vi "PH_BackreflectionMeas.ProcCases.vi"(0 "i ref in":refnum<vi>, 1 "selector":string, 2 "Data":T1, 3 "call cluster":T2={"Object"="", "Selector"="", "CallType"=enum."synchronous", "Async Object"="", "Async Selector"="", "Data Descriptor"="", "Data"=[], "Error #"=0, "Expire"=0}, 5 "error in (no error)":errorcluster) -> (14 "i ref out":refnum<vi>, 17 "answer cluster":T2={"Object"="", "Selector"="", "CallType"=enum."synchronous", "Async Object"="", "Async Selector"="", "Data Descriptor"="", "Data"=[], "Error #"=0, "Expire"=0}, 19 "error out":errorcluster)   [LabVIEW 2014, in "PH_BackreflectionMeas.lvlib"]
doc: "This method is called by a process from within the default case in the event loop. The methods of a class that are linked to events will be called from THIS method. Add your code here."
uses:
  PH_BackreflectionMeas.lvlib
  CS_Core/CSSystem/CoreDefs/CoreDefs.call_type.ctl
  CS_Core/BaseProcess/BaseProcess.descriptor string definition.ctl
  CS_Core/CSSystem/CoreDefs/CoreDefs.rawDataType.ctl
  PH_Basics/PH_StatusHandler/PH_StatusHandler.Status.ctl
  CS_Core/CSSystem/CoreLib/CoreLib.string 2 byte array.vi
  CS_Core/BaseProcess/BaseProcess.lvlib
  CS_Core/CSSystem/CoreLib/CoreLib.lvlib
  CS_Core/CAEObj/CAEObj.lvlib
  PH_Basics/PH_PSDBWriter/PH_PSDBWriter.lvlib
  PH_Devices/PH_TKTDS-30xx/PH_TKTDS-30xx.lvlib
  PH_Basics/PH_StatusHandler/PH_StatusHandler.lvlib
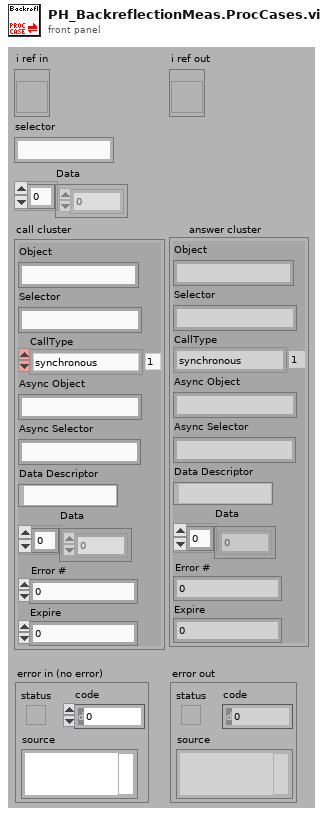
[diagram p1: front panel]
types:
  T1 = typedef "CoreDefs.rawDataType.ctl" = i8[]
  T2 = typedef "CoreDefs.call_type.ctl" = cluster{"Object":string, "Selector":string, "CallType":enum16{"simple", "synchronous", "asynchronous"}, "Async Object":string, "Async Selector":string, "Data Descriptor":T3, "Data":T1, "Error #":i32, "Expire":u32}
  T3 = typedef "BaseProcess.lvlib/BaseProcess.descriptor string definition.ctl" = string
  T4 = typedef "PH_StatusHandler.lvlib/PH_StatusHandler.Status.ctl" = i16
  T5 = typedef "PH_PSDBWriter.lvlib/PH_PSDBWriter.PHELIX-Subsystems.ctl" = i32
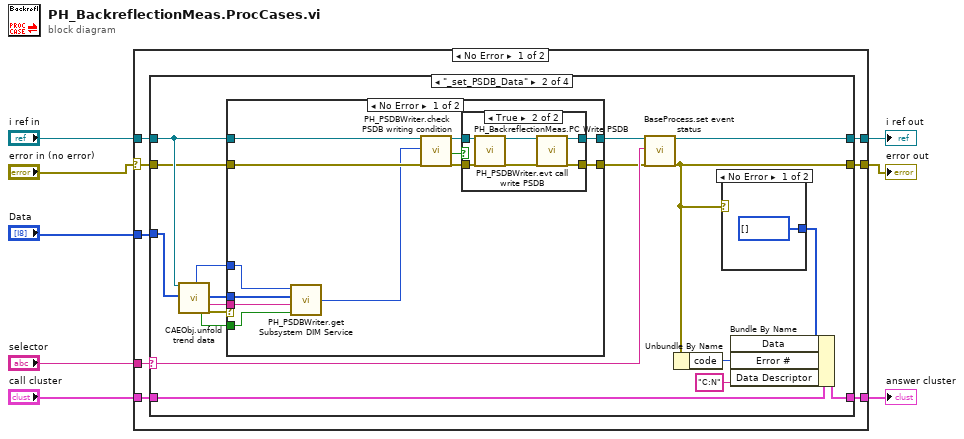
[diagram p0: block diagram]
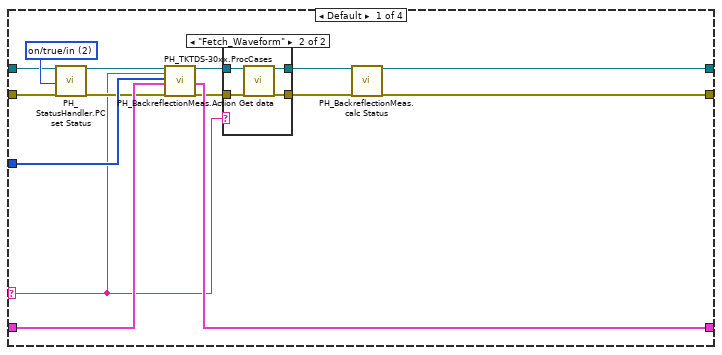
[diagram p2: hidden frame]
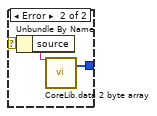
[diagram p6: hidden frame]
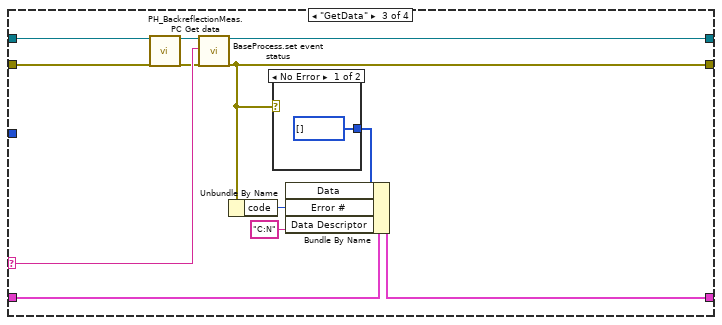
[diagram p7: hidden frame]
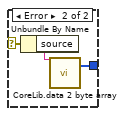
[diagram p8: hidden frame]
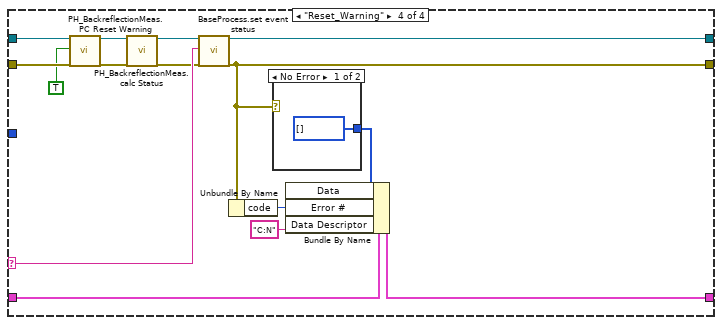
[diagram p9: hidden frame]
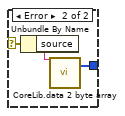
[diagram p10: hidden frame]
diagram:
  n1 = case shown="No Error" "error in (no error)" {
    selector: "error in (no error)" -> [w9 w117]
    tunnel: "selector" -> [w16 _]
    tunnel: [w15 w118] -> w7
    tunnel: "Data" -> [w14 _]
    tunnel: "call cluster" -> [w13 w118]
    tunnel: "i ref in" -> [w12 w119]
    tunnel: [w11 w119] -> w3
    tunnel: [w10 w117] -> w2
    frame No Error {
      n2 = case shown="\"_set_PSDB_Data\"" w16 {
        selector: w16 -> [w21 w50 w87 w106]
        tunnel: w14 -> [w29 w38 _ _]
        tunnel: w12 -> [w25 w42 w85 w104]
        tunnel: [w18 w49 w89 w108] -> w11
        tunnel: w13 -> [w30 w54 w86 w105]
        tunnel: [w31 w53 w92 w111] -> w15
        tunnel: w9 -> [w27 w40 w84 w103]
        tunnel: [w17 w51 w90 w109] -> w10
        frame Default {
          w28 = T4 2 items=["no info", "off/false/out", "on/true/in", "Failure", "Alarm", "Status 1", "Status 2", "Status 3"] ("Status")
          n3 = call "PH_StatusHandler.PC set Status.vi"("i ref in"=w25, "Status"=w28, "error in (no error)"=w27) -> ("i ref out"=w24:refnum<vi>, "error out"=w26:errorcluster)  [unwired: 15 in]
          n4 = call "PH_TKTDS-30xx.ProcCases.vi"("i ref in"=w24, "selector"=w21, "Data"=w29, "call cluster"=w30, "error in (no error)"=w26) -> ("i ref out"=w23:refnum<vi>, "answer cluster"=w31:T2, "error out"=w22:errorcluster)  [unwired: 12 in]
          n5 = case shown="\"Fetch_Waveform\"" w21 {
            tunnel: w23 -> [w33 w37]
            tunnel: [w33 w36] -> w19
            tunnel: w22 -> [w32 w35]
            tunnel: [w32 w34] -> w20
            frame Default {
            }
            frame "Fetch_Waveform" {
              n6 = call "PH_BackreflectionMeas.Action Get data.vi"("i ref in"=w37, "error IO"=w35) -> ("i ref out"=w36:refnum<vi>, "error out"=w34:errorcluster)  [unwired: 16 in]
            }
          }
          n7 = call "PH_BackreflectionMeas.calc Status.vi"("i ref in"=w19, "error in"=w20) -> ("i ref out"=w18:refnum<vi>, "error out"=w17:errorcluster)  [unwired: 16 in]
        }
        frame "_set_PSDB_Data" {
          n8 = call "CAEObj.unfold trend data.vi"("i ref in"=w42, "raw trend data"=w38) -> ("quality"=w43:i32, "no link"=w46:bool, "data"=w44:i8[], "typeDescriptor"=w45:string, "error out"=w47:errorcluster)  [unwired: 9 in, 4 out]
          n9 = case shown="No Error" w47 {
            tunnel: w40 -> [w67 w77]
            tunnel: [w66 w76] -> w41
            tunnel: [w65 w77] -> w39
            tunnel: w42 -> [w63 w76]
            tunnel: w46 -> [w57 _]
            tunnel: w45 -> [w59 _]
            tunnel: w44 -> [w60 _]
            tunnel: w43 -> [w58 _]
            frame No Error {
              n10 = call "PH_PSDBWriter.get Subsystem DIM Service.vi"("no link"=w57, "typeDescriptor"=w59, "data"=w60, "quality"=w58) -> ("PHELIX Subsystems"=w56:T5)
              n11 = call "PH_PSDBWriter.check PSDB writing condition.vi"("i ref in"=w63, "wanted Subsystem"=w56, "error IO"=w67) -> ("i ref out"=w62:refnum<vi>, "write PSDB?"=w61:bool, "error out"=w64:errorcluster)  [unwired: 14 in]
              n12 = case shown="True" w61 {
                tunnel: w64 -> [w68 w75]
                tunnel: [w69 w72] -> w66
                tunnel: [w68 w70] -> w65
                tunnel: w62 -> [w69 w74]
                frame False {
                }
                frame True {
                  n13 = call "PH_BackreflectionMeas.PC Write PSDB.vi"("i ref in"=w74, "error IO"=w75) -> ("i ref out"=w73:refnum<vi>, "error out"=w71:errorcluster)  [unwired: 16 in]
                  n14 = call "PH_PSDBWriter.evt call write PSDB.vi"("i ref in"=w73, "error in (no error)"=w71) -> ("i ref out"=w72:refnum<vi>, "error out"=w70:errorcluster)  [unwired: 16 in]
                }
              }
            }
            frame Error {
            }
          }
          n15 = call "BaseProcess.set event status.vi"("i ref in"=w41, "EventStatus"=w50, "error in (no error)"=w39) -> ("i ref out"=w49:refnum<vi>, "error out"=w51:errorcluster)  [unwired: 14 in, 1 out]
          n16 = Unbundle By Name(w51) -> ("code"=w55:i32)
          n17 = case shown="No Error" w51 {
            selector: w51 -> [_ w81]
            tunnel: [T1 [] ("byteArray out") w80] -> w52
            frame No Error {
            }
            frame Error {
              n18 = Unbundle By Name(w81) -> ("source"=w79:string)
              n19 = call-poly "CoreLib.data 2 byte array.vi"("string"=w79) -> ("byteArray out"=w80:T1)  [unwired: 18 in]
            }
          }
          n20 = Bundle By Name(cluster=w54, "Data"=w52, "Error #"=w55, "Data Descriptor"="C:N") -> (w53:T2)
        }
        frame "GetData" {
          n21 = call "PH_BackreflectionMeas.PC Get data.vi"("i ref in"=w85, "error IO"=w84) -> ("i ref out"=w83:refnum<vi>, "error out"=w82:errorcluster)  [unwired: 16 in]
          n22 = call "BaseProcess.set event status.vi"("i ref in"=w83, "EventStatus"=w87, "error in (no error)"=w82) -> ("i ref out"=w89:refnum<vi>, "error out"=w90:errorcluster)  [unwired: 14 in, 1 out]
          n23 = Unbundle By Name(w90) -> ("code"=w93:i32)
          n24 = case shown="No Error" w90 {
            selector: w90 -> [_ w97]
            tunnel: [T1 [] ("byteArray out") w96] -> w91
            frame No Error {
            }
            frame Error {
              n25 = Unbundle By Name(w97) -> ("source"=w95:string)
              n26 = call-poly "CoreLib.data 2 byte array.vi"("string"=w95) -> ("byteArray out"=w96:T1)  [unwired: 18 in]
            }
          }
          n27 = Bundle By Name(cluster=w86, "Data"=w91, "Error #"=w93, "Data Descriptor"="C:N") -> (w92:T2)
        }
        frame "Reset_Warning" {
          n28 = call "PH_BackreflectionMeas.PC Reset Warning.vi"("i ref in"=w104, "Reset Warning?"=TRUE, "error in (no error)"=w103) -> ("i ref out"=w101:refnum<vi>, "error out"=w99:errorcluster)  [unwired: 15 in]
          n29 = call "PH_BackreflectionMeas.calc Status.vi"("i ref in"=w101, "error in"=w99) -> ("i ref out"=w100:refnum<vi>, "error out"=w98:errorcluster)  [unwired: 16 in]
          n30 = call "BaseProcess.set event status.vi"("i ref in"=w100, "EventStatus"=w106, "error in (no error)"=w98) -> ("i ref out"=w108:refnum<vi>, "error out"=w109:errorcluster)  [unwired: 14 in, 1 out]
          n31 = Unbundle By Name(w109) -> ("code"=w112:i32)
          n32 = case shown="No Error" w109 {
            selector: w109 -> [_ w116]
            tunnel: [T1 [] ("byteArray out") w115] -> w110
            frame No Error {
            }
            frame Error {
              n33 = Unbundle By Name(w116) -> ("source"=w114:string)
              n34 = call-poly "CoreLib.data 2 byte array.vi"("string"=w114) -> ("byteArray out"=w115:T1)  [unwired: 18 in]
            }
          }
          n35 = Bundle By Name(cluster=w105, "Data"=w110, "Error #"=w112, "Data Descriptor"="C:N") -> (w111:T2)
        }
      }
    }
    frame Error {
    }
  }
  "answer cluster" <- w7
  "i ref out" <- w3
  "error out" <- w2
